vi "Get_File_Info_Listing.vi"(0 "path":path) -> (1 "Path":path[](array[path]), 2 "Last Mod":dbl[](array[numeric]), 3 "Size":i64[](array[numeric]))   [LabVIEW 2018]
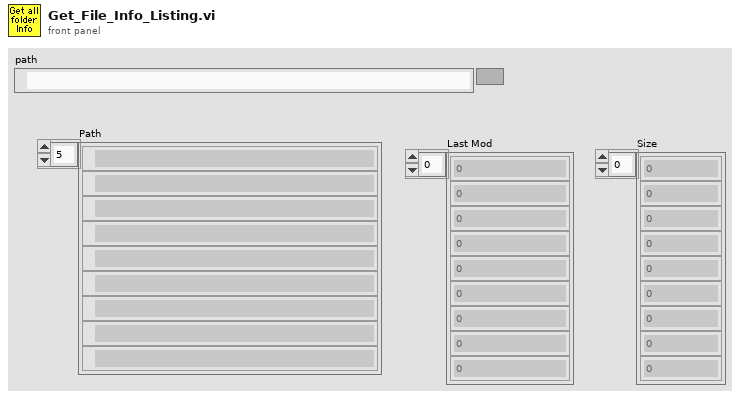
[diagram p1: front panel]
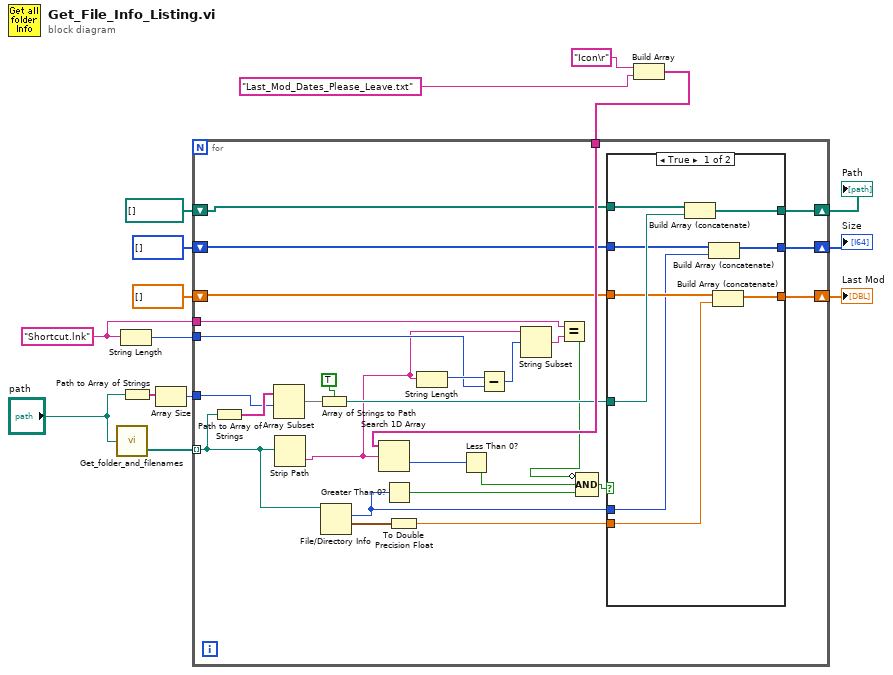
[diagram p0: block diagram]
diagram:
  w1 = "Shortcut.lnk"
  n1 = call "Get_folder_and_filenames.vi"("file path (dialog if empty)"="path") -> ("Files"=w11:path[])  [unwired: 1 out]
  n2 = String Length(string=w1) -> (length=w2:i32)
  n3 = Path to Array of Strings(0:"path") -> (2:w12:string[])  [unwired: 1 out]
  n4 = Array Size(array=w12) -> (size(s)=w13:i32)
  n5 = Build Array("Icon\r", "Last_Mod_Dates_Please_Leave.txt" ("name or relative path")) -> (w15:string[])
  n6 = for {
    tunnel: w11 -> [w30] mode=indexing
    tunnel: w13 -> [w41]
    shift-right: [w35] -> w5
    shift-left: path[] [] -> [w36]
    tunnel: w15 -> [w40]
    shift-right: [w33] -> w6
    shift-left: i64[] [] -> [w34]
    shift-right: [w31] -> w7
    shift-left: dbl[] [] -> [w32]
    tunnel: w2 -> [w21]
    tunnel: w1 -> [w18]
    n7 = Path to Array of Strings(0:w30) -> (2:w42:string[])  [unwired: 1 out]
    n8 = Array Subset(array=w42, index=w41) -> (w38:string[])  [unwired: 1 in]
    n9 = Strip Path(path=w30) -> (name=w16:string)  [unwired: 1 out]
    n10 = Array of Strings to Path(0:w38, 1:TRUE ("relative")) -> (2:w23:path)
    n11 = File/Directory Info(path=w30) -> (size=w26:i64, last mod=w25:timestamp)  [unwired: 1 in, 5 out]
    n12 = Search 1D Array(1D array=w40, element=w16) -> (index of element=w39:i32)  [unwired: 1 out]
    n13 = Greater Than 0?(x=w26) -> (x > 0?=w28:bool)
    n14 = To Double Precision Float(number=w25) -> (double precision float=w24:dbl)
    n15 = String Length(string=w16) -> (length=w22:i32)
    n16 = Less Than 0?(x=w39) -> (x < 0?=w29:bool)
    n17 = Subtract(x=w22, y=w21) -> (x-y=w20:i32)
    n18 = String Subset(string=w16, offset (0)=w20) -> (substring=w19:string)  [unwired: 1 in]
    n19 = Equal?(x=w18, y=w19) -> (x = y?=w17:bool)
    n20 = Compound Arithmetic op=AND(invert w17, w29, w28) -> (w27:bool)
    n21 = case shown="True" w27 {
      tunnel: w36 -> [w51 w54]
      tunnel: w23 -> [w50 _]
      tunnel: [w49 w54] -> w35
      tunnel: w34 -> [w48 w53]
      tunnel: [w47 w53] -> w33
      tunnel: w32 -> [w46 w52]
      tunnel: [w45 w52] -> w31
      tunnel: w24 -> [w44 _]
      tunnel: w26 -> [w43 _]
      frame True {
        n22 = Build Array (concatenate)(w51, w50) -> (w49:path[])
        n23 = Build Array (concatenate)(w48, w43) -> (w47:i64[])
        n24 = Build Array (concatenate)(w46, w44) -> (w45:dbl[])
      }
      frame False {
      }
    }
  }
  "Last Mod" <- w7
  "Size" <- w6
  "Path" <- w5
